vi "Configure Macro Execution State.vi"(8 "error in (no error)":errorcluster, 10 "Macro Execution State (Off)":bool, 11 "VISA resource name":refnum<visa-resource-name>) -> (0 "error out":errorcluster, 3 "VISA resource name out":refnum<visa-resource-name>)   [LabVIEW 2020, in "Rohde&Schwarz CMXP Base.lvlib"]
doc: "Enables or disables the execution of all macros that are defined for the active remote connection. Note: In contrast to SCPI specifications, macro execution is disabled by default.\n\nAttribute:\nRSCMXPBASE_ATTR_MACRO_EXECUTION_STATE\n\nRemote-control command:\n*EMC"
uses:
  <instrlib>/Rohde&Schwarz CMXP Base/Rohde&Schwarz CMXP Base.lvlib
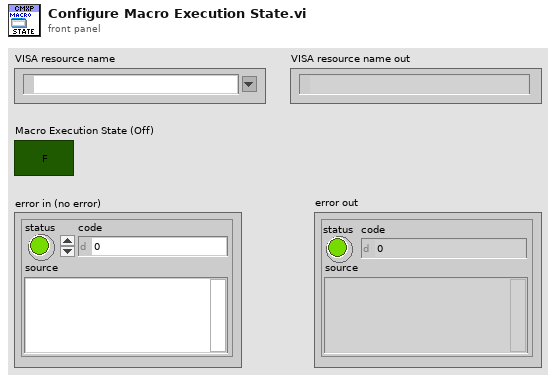
[diagram p1: front panel]
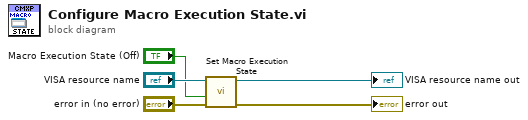
[diagram p0: block diagram]
diagram:
  n1 = call "Set Macro Execution State"("error in (no error)"="error in (no error)", "Macro Execution State (OFF)"="Macro Execution State (Off)", "instrument handle"="VISA resource name") -> ("error out"=→"error out":errorcluster, "instrument handle out"=→"VISA resource name out":refnum<visa-resource-name>)  [unwired: 7 in]
